vi "print test.vi"(0 "Data to Printer":string[](array[string]), 5 "Printer Port":refnum<visa-resource-name>="COM1") -> (4 "Write Data":string="﻿\u0010CT~~CD,~CC^~CT~\n^XA~TA000~JSN^LT0^MNW^MTD^PON^PMN^LH0,0^JMA^PR4,4~SD30^JUS^LRN^CI0^XZ\n~DG000.GRF,01024,016,\n,:::::::::::::::::::M02,M03F8,M03E0,:M03E0R020,M03F80P07C0,M03080P0F,M03080P07,M021867FBFE7F9FDFCFFBFF3FC0M02186618E061DC07003BC730C0N0386618E061D807003B8730C0N0386618E07FD8070FDB803FC0N0786618E06018070C3B8030,M03F86618FE7FD8070FFBFF3FC0M03F866187E7FD8070FF9FF3FC0,::::::::::::::::::::::::::::^XA\n^MMT\n^PW318\n^LL0128\n^LS0\n^FT80,78^A0N,14,12^FH\\^FD09/08/14^FS\n^FT0,128^XG000.GRF,1,1^FS\n^FT77,36^A0N,14,14^FH\\^FDLEDMAK^FS\n^FT35,78^A0N,14,14^FH\\^FD11111^FS\n^FT42,57^A0N,14,14^FH\\^FDBA^FS\n^FT93,57^A0N,14,14^FH\\^FD34^FS\n^FT34,36^A0N,14,14^FH\\^FDW105^FS\n^FO28,81^GB101,0,2^FS\n^FO26,61^GB103,0,2^FS\n^FO25,18^GB106,86,2^FS\n^FO27,40^GB103,0,2^FS\n^FO73,19^GB0,63,1^FS\n^FT142,114^BQN,2,3\n^FDMA,700222662X-6240908201402A12345XXX0001BCAV4FS001T001^FS\n^PQ1,0,1,Y^XZ\n^XA^ID000.GRF^FS^XZ\n")   [LabVIEW 2015]
panel:
  in  "LABEl":string="<xpml><page quantity='0' pitch='27.9 mm'></xpml>'Seagull:2.1:DP\nINPUT OFF\nVERBOFF\nINPUT ON\nSYSVAR(48) = 0\nERROR 15,\"FONT NOT FOUND\"\nERROR 18,\"DISK FULL\"\nERROR 26,\"PARAMETER TOO LARGE\"\nERROR 27,\"PARAMETER TOO SMALL\"\nERROR 37,\"CUTTER DEVICE NOT FOUND\"\nERROR 1003,\"FIELD OUT OF LABEL\"\nSYSVAR(35)=0\nOPEN \"tmp:setup.sys\" FOR OUTPUT AS #1\nPRINT#1,\"Printing,Media,Print Area,Media Margin (X),0\"\nPRINT#1,\"Printing,Media,Clip Default,On\"\nCLOSE #1\nSETUP \"tmp:setup.sys\"\nKILL \"tmp:setup.sys\"\n<xpml></page></xpml><xpml><page quantity='1' pitch='27.9 mm'></xpml>CLL\nOPTIMIZE \"BATCH\" ON\nPP249,177:AN7\nBARSET \"DATAMATRIX\",1,1,5,90,0,5\nPB \"B093285002M65M40-LH300318\"\nPP33,190:NASC 8\nFT \"Andale Mono Bold\",11,0,75\nPT \"85051M85M60-BFB\"\nPP32,99:FT \"Andale Mono Bold\",11,0,43\nPT \"A093285002M65M40-LH300318\"\nLAYOUT RUN \"\"\nPF\nPRINT KEY OFF\n<xpml></page></xpml><xpml><end/></xpml>"
  out "x = y?":bool
  out "Read  Data":string="﻿\u0010CT~~CD,~CC^~CT~\n^XA~TA000~JSN^LT0^MNW^MTD^PON^PMN^LH0,0^JMA^PR4,4~SD30^JUS^LRN^CI0^XZ\n~DG000.GRF,01024,016,\n,:::::::::::::::::::M02,M03F8,M03E0,:M03E0R020,M03F80P07C0,M03080P0F,M03080P07,M021867FBFE7F9FDFCFFBFF3FC0M02186618E061DC07003BC730C0N0386618E061D807003B8730C0N0386618E07FD8070FDB803FC0N0786618E06018070C3B8030,M03F86618FE7FD8070FFBFF3FC0M03F866187E7FD8070FF9FF3FC0,::::::::::::::::::::::::::::^XA\n^MMT\n^PW318\n^LL0128\n^LS0\n^FT80,78^A0N,14,12^FH\\^FD09/08/14^FS\n^FT0,128^XG000.GRF,1,1^FS\n^FT77,36^A0N,14,14^FH\\^FDLAE67F^FS\n^FT35,78^A0N,14,14^FH\\^FD99999^FS\n^FT42,57^A0N,14,14^FH\\^FDCB^FS\n^FT93,57^A0N,14,14^FH\\^FD34^FS\n^FT34,36^A0N,14,14^FH\\^FDW105^FS\n^FO28,81^GB101,0,2^FS\n^FO26,61^GB103,0,2^FS\n^FO25,18^GB106,86,2^FS\n^FO27,40^GB103,0,2^FS\n^FO73,19^GB0,63,1^FS\n^FT142,114^BQN,2,3\n^FDMA,700222662X-6240908201402A12345XXX0001BCAV4FS001T001^FS\n^PQ1,0,1,Y^XZ\n^XA^ID000.GRF^FS^XZ\n"
  # "86751-82R00/85051M65MA0-CW8/16"
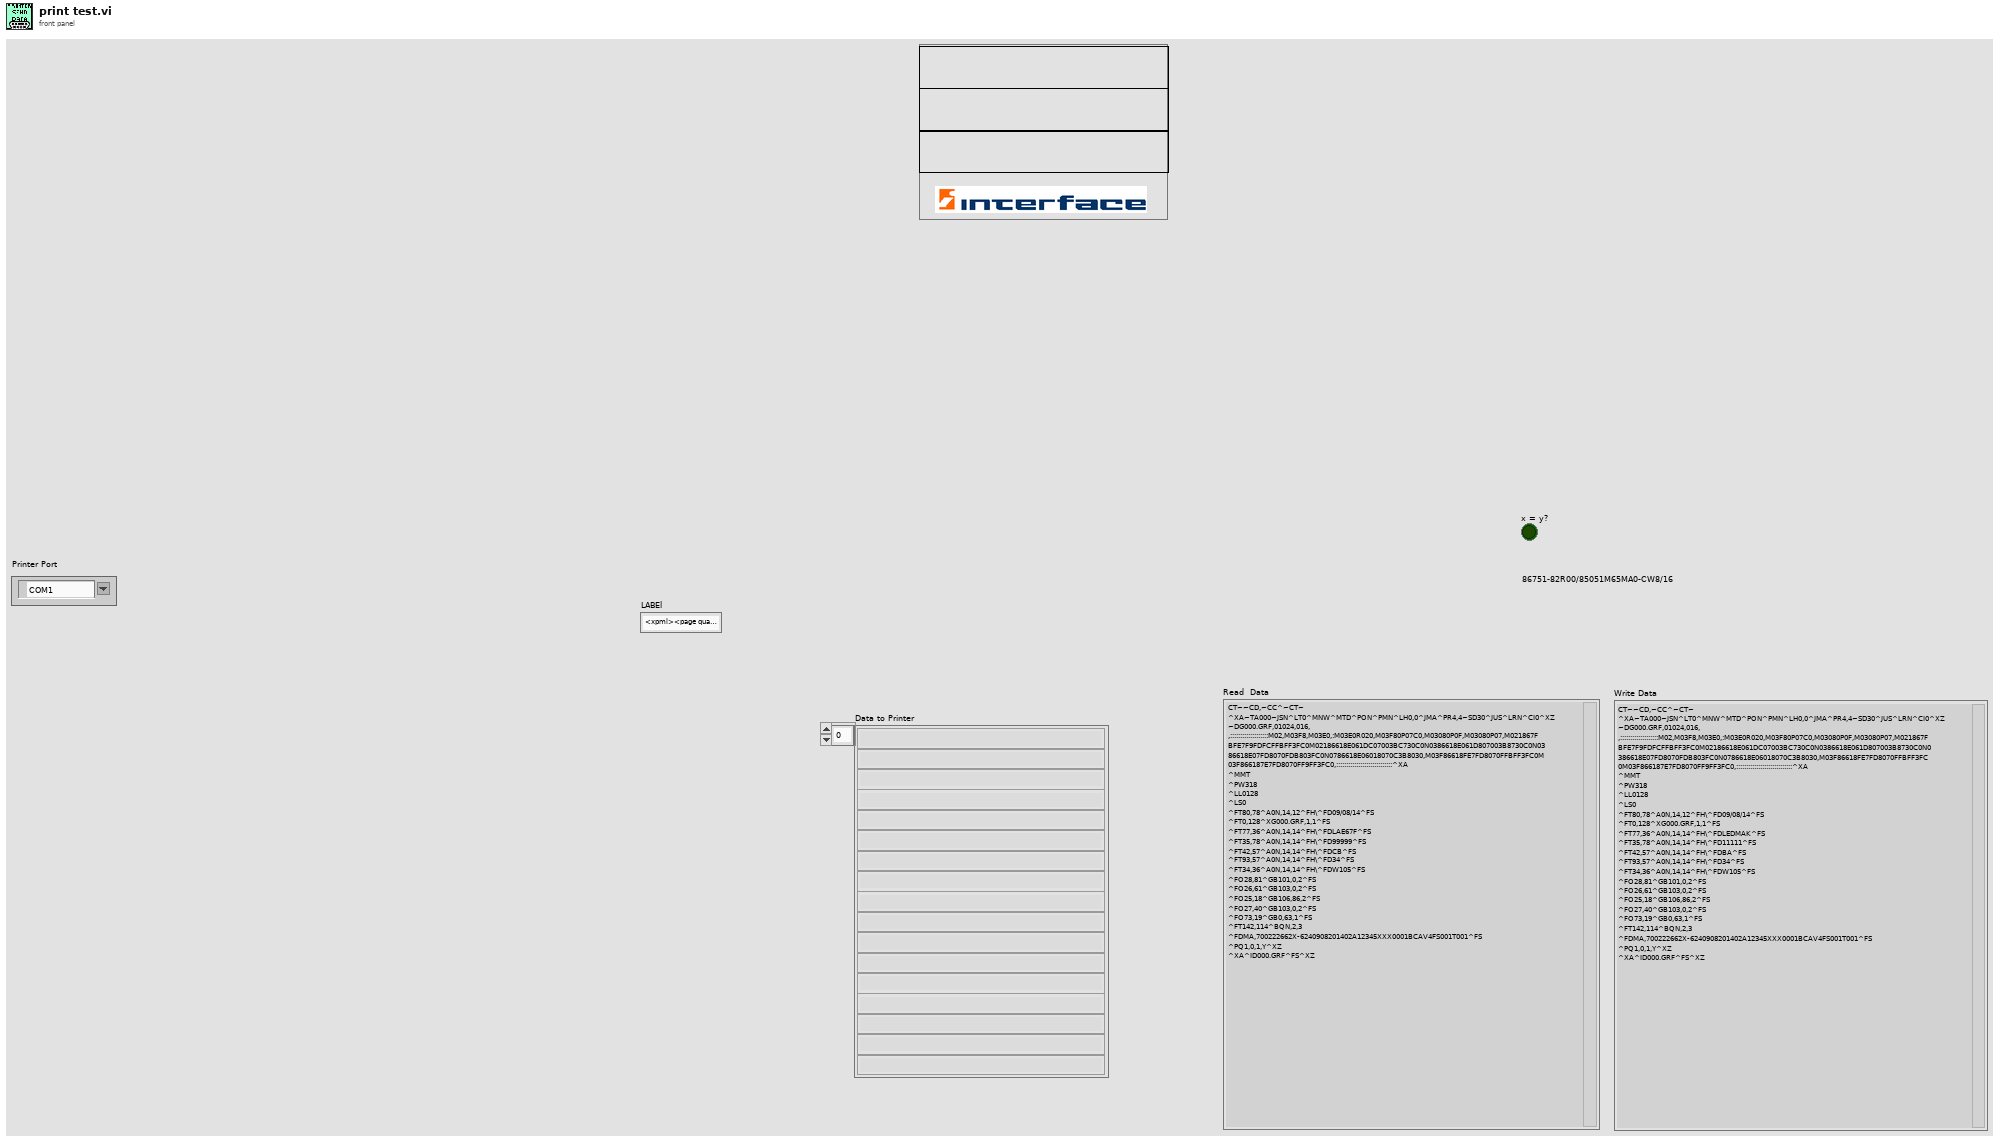
[diagram p1: front panel]
types:
  T1 = enum16{"open", "replace", "create", "open or create", "replace or create", "replace or create with confirmation"}
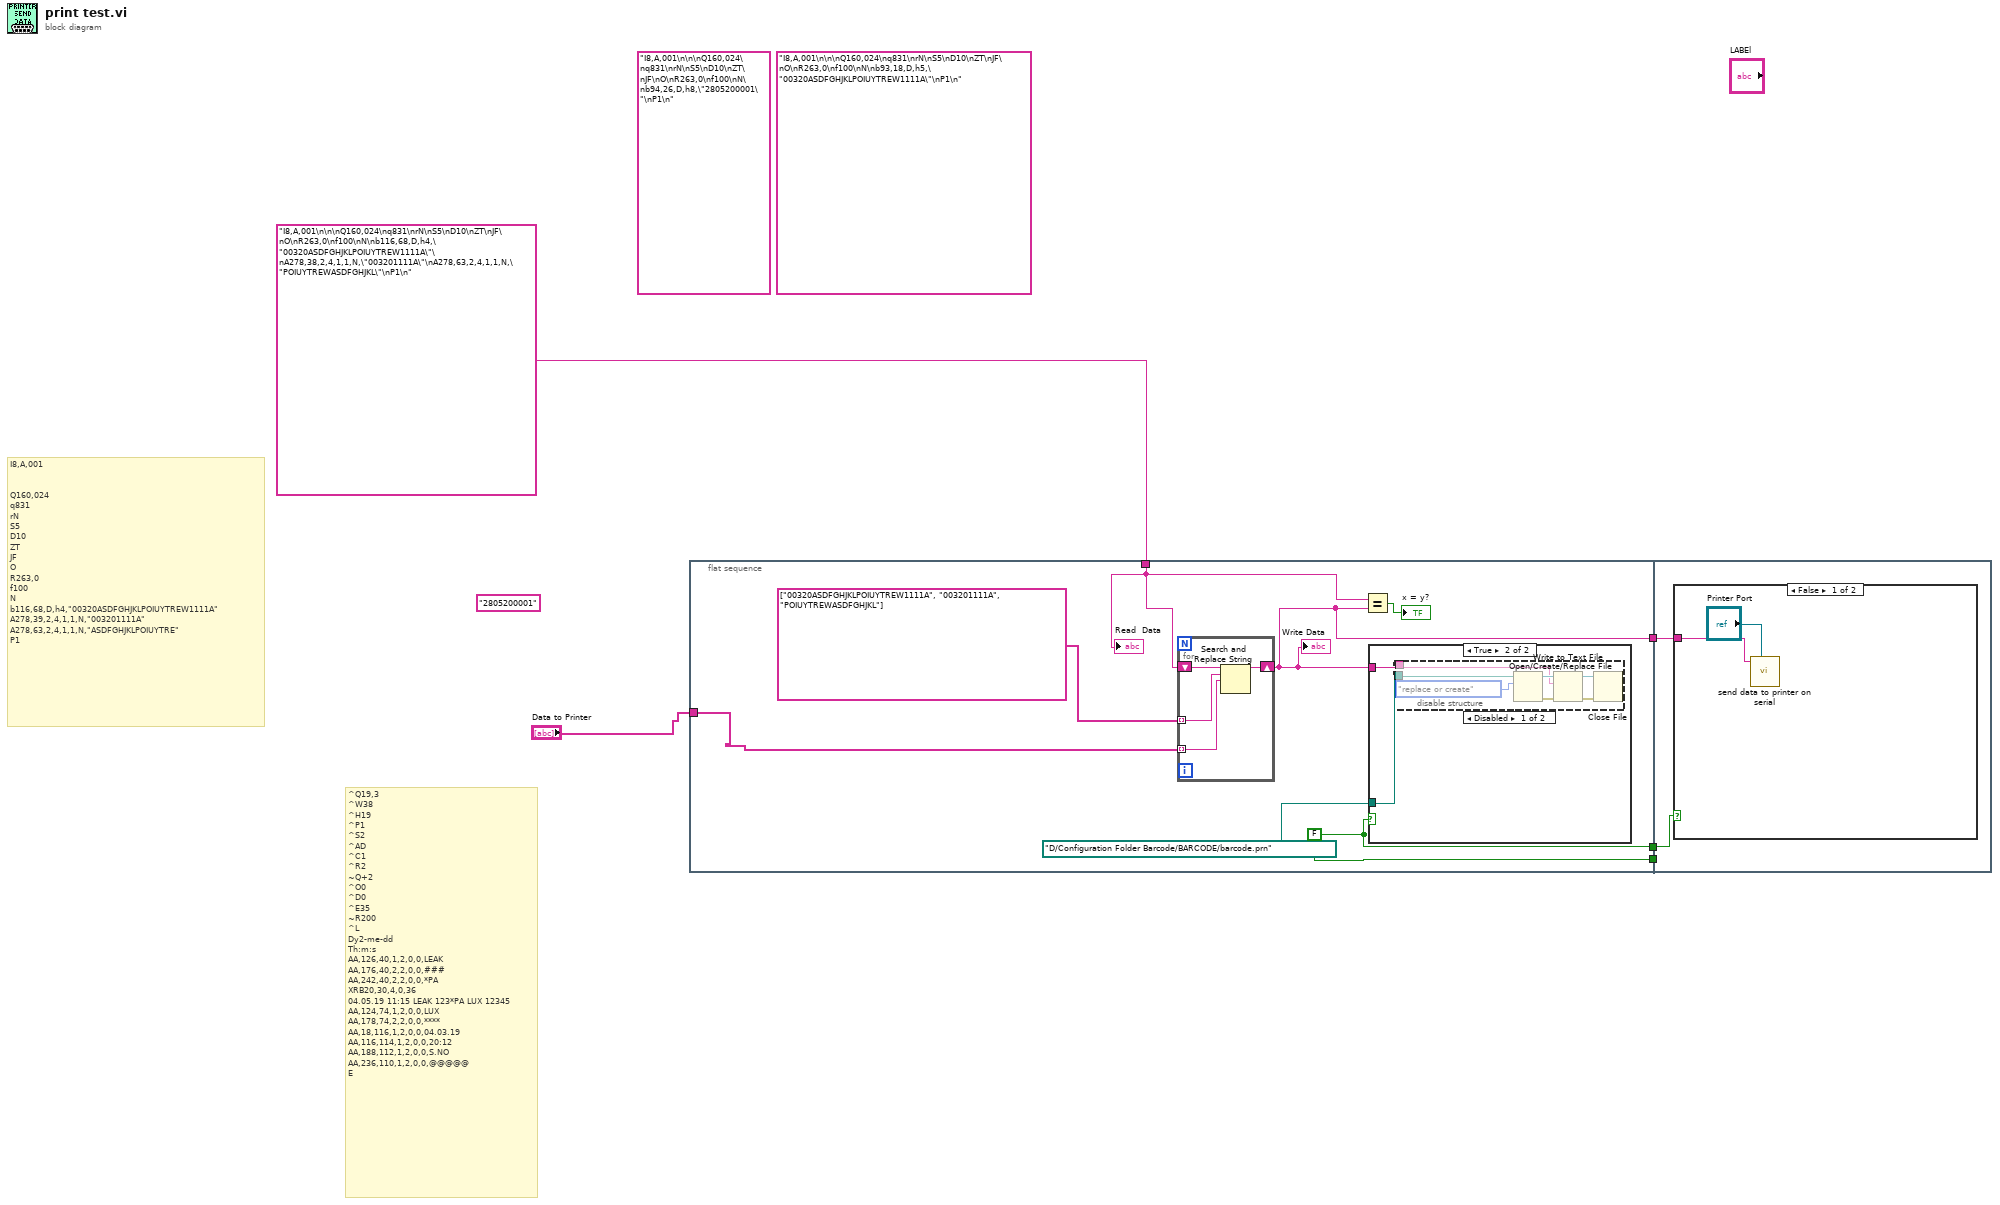
[diagram p0: block diagram]
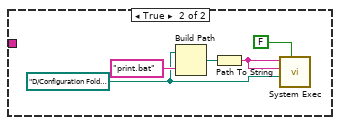
[diagram p4: hidden frame]
diagram:
  (unwired) "I8,A,001\n\n\nQ160,024\nq831\nrN\nS5\nD10\nZT\nJF\nO\nR263,0\nf100\nN\nb94,26,D,h8,\"2805200001\"\nP1\n"
  (unwired) "I8,A,001\n\n\nQ160,024\nq831\nrN\nS5\nD10\nZT\nJF\nO\nR263,0\nf100\nN\nb93,18,D,h5,\"00320ASDFGHJKLPOIUYTREW1111A\"\nP1\n"
  (unwired) "2805200001" ("Vender Code")
  # "I8,A,001\n\n\nQ160,024\nq831\nrN\nS5\nD10\nZT\nJF\nO\nR263,0\nf100\nN\nb116,68,D,h4,\"00320ASDFGHJKLPOIUYTREW1111A\"\nA278,39,2,4,1,1,N,\"003201111A\"\nA278,63,2,4,1,1,N,\"ASDFGHJKLPOIUYTRE\"\nP1"
  # "^Q19,3\n^W38\n^H19\n^P1\n^S2\n^AD\n^C1\n^R2\n~Q+2\n^O0\n^D0\n^E35\n~R200\n^L\nDy2-me-dd\nTh:m:s\nAA,126,40,1,2,0,0,LEAK\nAA,176,40,2,2,0,0,###\nAA,242,40,2,2,0,0,*PA\nXRB20,30,4,0,36\n04.05.19 11:15 LEAK 123*PA LUX 12345\nAA,124,74,1,2,0,0,LUX\nAA,178,74,2,2,0,0,****\nAA,18,116,1,2,0,0,04.03.19\nAA,116,114,1,2,0,0,20:12\nAA,188,112,1,2,0,0,S.NO\nAA,236,110,1,2,0,0,@@@@@\nE"
  n1 = flat-sequence {
    tunnel: [w12] -> w5
    tunnel: [w12] -> w4
    tunnel: "I8,A,001\n\n\nQ160,024\nq831\nrN\nS5\nD10\nZT\nJF\nO\nR263,0\nf100\nN\nb116,68,D,h4,\"00320ASDFGHJKLPOIUYTREW1111A\"\nA278,38,2,4,1,1,N,\"003201111A\"\nA278,63,2,4,1,1,N,\"POIUYTREWASDFGHJKL\"\nP1\n" -> [w8]
    tunnel: [w7] -> w2
    tunnel: "Data to Printer" -> [w6]
    tunnel: w5 -> [_]
    tunnel: w4 -> [w27]
    tunnel: w2 -> [w26]
    frame #0 {
      w12 = FALSE ("Print")
      n2 = for {
        shift-right: [w25] -> w7
        shift-left: w8 -> [w24]
        tunnel: w6 -> [w22] mode=indexing
        tunnel: string[] ["00320ASDFGHJKLPOIUYTREW1111A", "003201111A", "POIUYTREWASDFGHJKL"] ("array 2") -> [w23] mode=indexing
        n3 = Search and Replace String(input string=w24, search string=w23, replace string=w22) -> (result string=w25:string)  [unwired: 5 in, 3 out]
      }
      "Write Data" <- w7
      n4 = Equal?(x=w8, y=w7) -> (x = y?=→"x = y?":bool)
      n5 = case shown="True" w12 {
        tunnel: w7 -> [_ w14]
        tunnel: path "D:/Configuration Folder Barcode/BARCODE/barcode.prn" ("file path (use dialog)") -> [_ w13]
        frame False {
        }
        frame True {
          n6 = disable-structure shown="Disabled" {
            disable-tunnel: w14 -> [w17 _]
            disable-tunnel: w13 -> [w16 _]
            frame Disabled {
              n7 = Open/Create/Replace File(file path (use dialog)=w16, operation (0:open)=T1."replace or create") -> (refnum out=w21:refnum<file>, error out=w20:errorcluster)  [unwired: 4 in, 1 out]
              n8 = Write to Text File(file (use dialog)=w21, text=w17, error in=w20) -> (refnum out=w18:refnum<file>, error out=w19:errorcluster)  [unwired: 1 in, 1 out]
              n9 = Close File(refnum=w18, error in=w19) -> ()  [unwired: 2 out]
            }
            frame Enabled {
            }
          }
        }
      }
      "Read  Data" <- w8
    }
    frame #1 {
      n10 = case shown="False" w27 {
        tunnel: w26 -> [w29 _]
        frame False {
          n11 = call "send data to printer on serial.vi"("VISA resource name"="Printer Port", "Command"=w29) -> ()  [unwired: 10 in]
        }
        frame True {
          w32 = path "D:/Configuration Folder Barcode/BARCODE" ("working directory")
          n12 = Build Path(base path=w32, name or relative path="print.bat") -> (appended path=w31:path)
          n13 = Path To String(path=w31) -> (string=w30:string)
          n14 = call <vilib>:"System Exec.vi"("wait until completion? (T)"=FALSE, "working directory"=w32, "standard input"=w30, "command line"=w30) -> ()  [unwired: 4 in, 4 out]
        }
      }
    }
  }
